vi "Profile Auton - Intake.vi"(7 "error in (no error)":errorcluster, 9 "Time (s)":dbl, 10 "Intake":bool) -> (0 "error out":errorcluster)   [LabVIEW 2017]
uses:
  Robot Global Data.vi
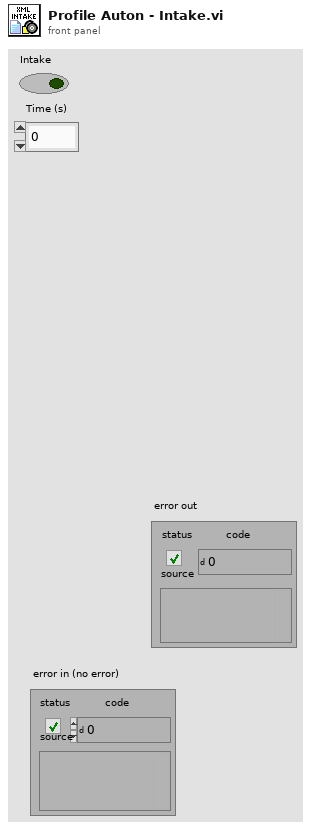
[diagram p1: front panel]
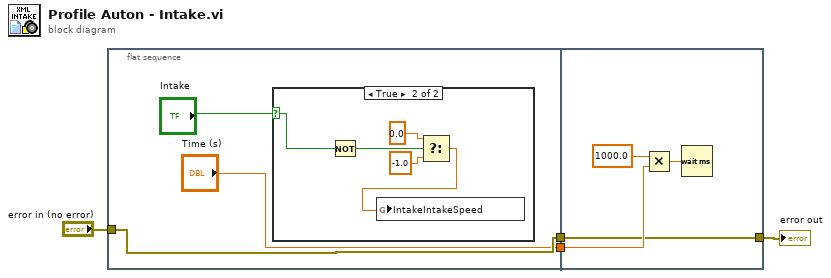
[diagram p0: block diagram]
diagram:
  n1 = flat-sequence {
    tunnel: ["Time (s)"] -> w4
    tunnel: [w7] -> w2
    tunnel: "error in (no error)" -> [w7]
    tunnel: w4 -> [w15]
    tunnel: [w13] -> w3
    tunnel: w2 -> [w13]
    frame #0 {
      n2 = case shown="True" "Intake" {
        selector: "Intake" -> [_ w10]
        frame False {
        }
        frame True {
          n3 = Not(x=w10) -> (.not. x?=w9:bool)
          n4 = Select(t=0.0, s=w9, f=-1.0 ("t")) -> (s? t:f=w8:dbl)
          n5 = global write "Robot Global Data.vi" "IntakeIntakeSpeed"(w8) -> ()
        }
      }
    }
    frame #1 {
      n6 = Multiply(x=1000.0, y=w15) -> (x*y=w16:dbl)
      n7 = Wait (ms)(milliseconds to wait=w16) -> ()  [unwired: 1 out]
    }
  }
  "error out" <- w3
